vi "BuildDecisionTree_alt.vi"(8 "error in (no error)":errorcluster, 9 "Current Player":T1=enum."Player 1", 10 "Gameboard":T2=[enum."None", enum."None", enum."None", enum."None", enum."None", enum."None", enum."None", enum."None", enum."None"], 11 "DecisionTree In":T3) -> (0 "error out":errorcluster, 2 "Status":T1, 3 "DecisionTree Out":T3)   [LabVIEW 2020]
uses:
  controls/DecisionTree.ctl
  controls/Gameboard Data.ctl
  controls/DecisionTreeRecord.ctl
  controls/Player.ctl
  GetEquivalentKeysNumeric.vi
  AllLines.vi
  MakeSquare.vi
  Flatten2DArray.vi
  <vilib>/Utility/error.llb/Error Cluster From Error Code.vi
  GetAllIsometriesOf2DArray.vi
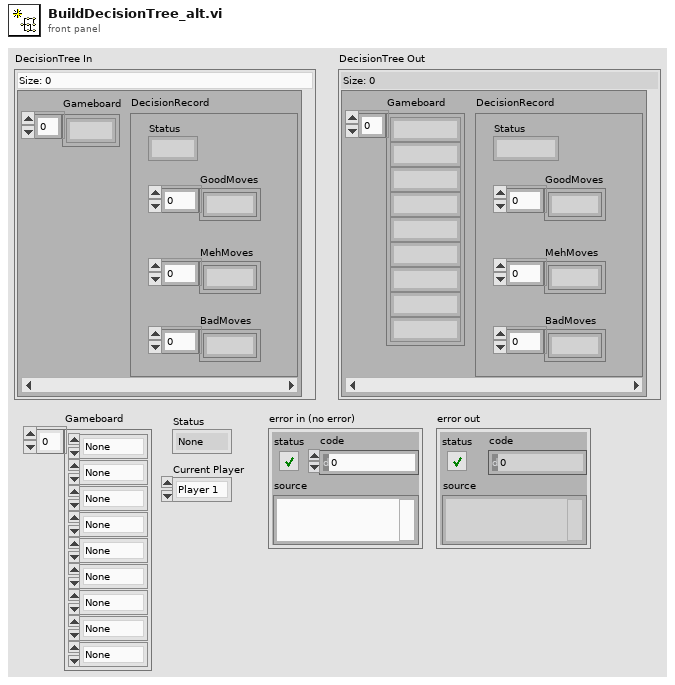
[diagram p1: front panel]
types:
  T1 = typedef "Player.ctl" = enum16{"None", "Player 1", "Player 2"}
  T2 = typedef "Gameboard Data.ctl" = enum16{"None", "Player 1", "Player 2"}[]
  T3 = typedef "DecisionTree.ctl" = map{T2, T4}
  T4 = typedef "DecisionTreeRecord.ctl" = cluster{"Status":T1, "GoodMoves":i8[], "MehMoves":i8[], "BadMoves":i8[]}
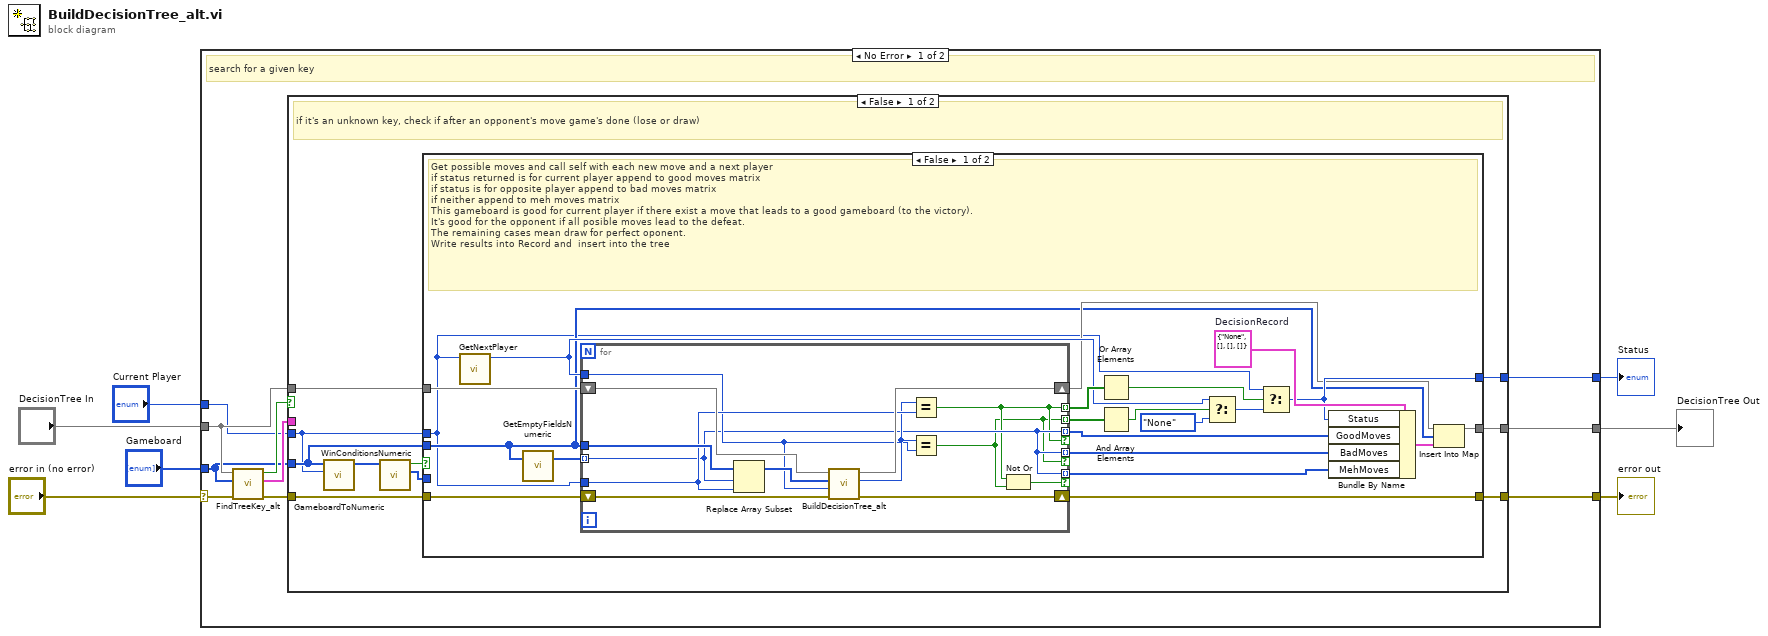
[diagram p0: block diagram]
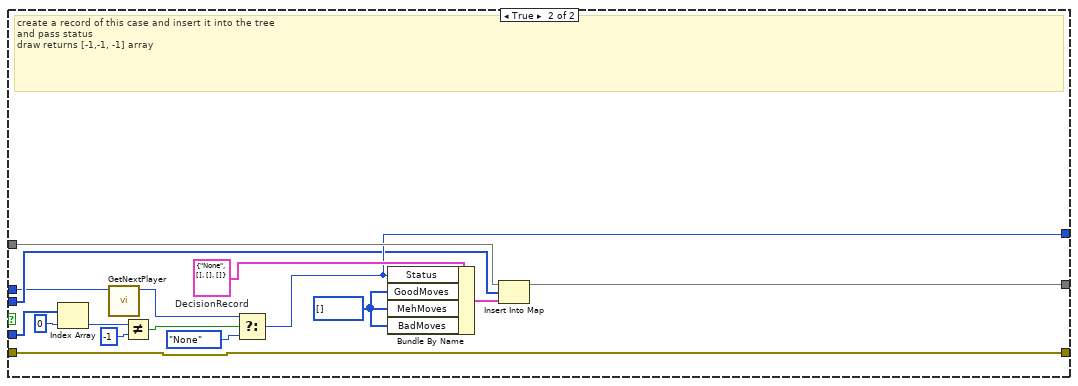
[diagram p2: hidden frame]
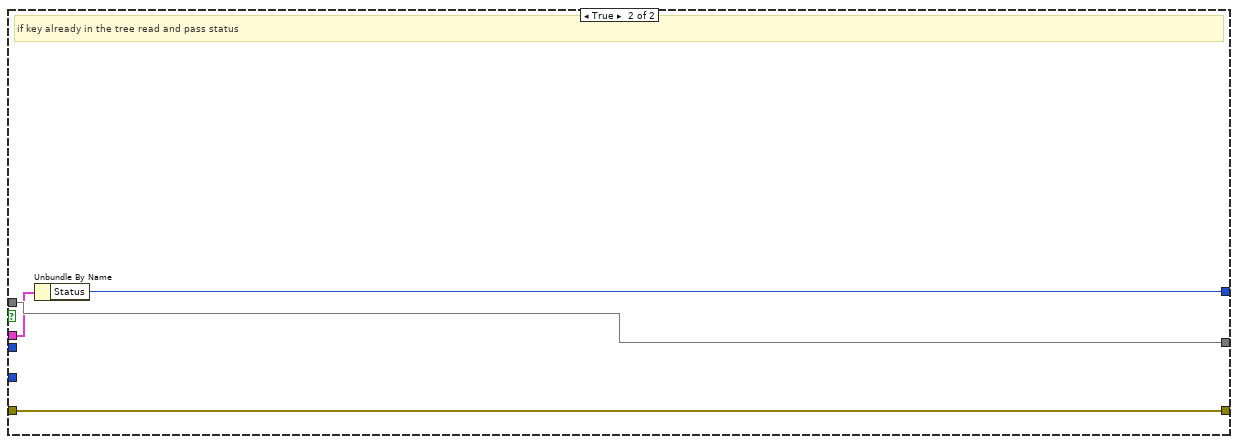
[diagram p3: hidden frame]
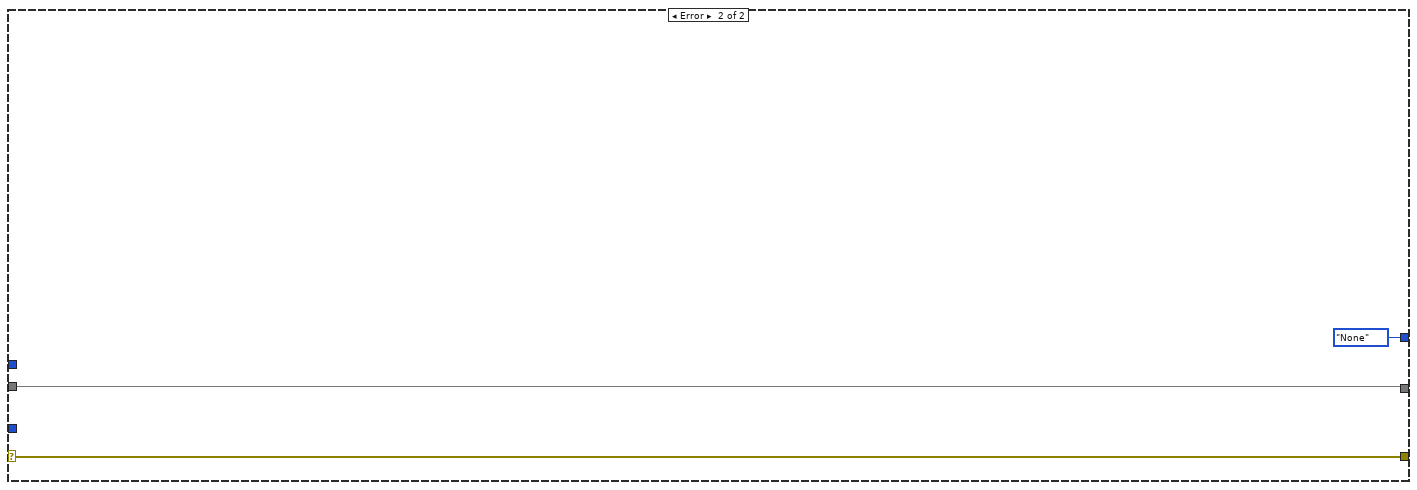
[diagram p4: hidden frame]
diagram:
  n1 = case shown="No Error" "error in (no error)" {
    selector: "error in (no error)" -> [w17 w84]
    tunnel: [w12 w84] -> w6
    tunnel: "Gameboard" -> [w9 _]
    tunnel: "Current Player" -> [w8 _]
    tunnel: [w10 Player."None" ("Status")] -> w3
    tunnel: "DecisionTree In" -> [w14 w82]
    tunnel: [w13 w82] -> w1
    frame No Error {
      # "search for a given key"
      n2 = call "FindTreeKey_alt.vi"("error in (no error)"=w17, "Key"=w9, "Map"=w14) -> ("error out"=w15:errorcluster, "DecisionRecord"=w11:T4, "IsFound?"=w16:bool)  [unwired: 5 in, 1 out]
      n3 = case shown="False" w16 {
        tunnel: w15 -> [w22 w80]
        tunnel: w14 -> [w21 w81]
        tunnel: [w20 w81] -> w13
        tunnel: [w18 w80] -> w12
        tunnel: w11 -> [_ w79]
        tunnel: [w19 w78] -> w10
        tunnel: w9 -> [w24 _]
        tunnel: w8 -> [w23 _]
        frame False {
          # "if it's an unknown key, check if after an opponent's move game's done (lose or draw)"
          n4 = call "GameboardToNumeric.vi"("CurrentPlayer"=w23, "Gameboard"=w24) -> ("NumericGameboard"=w25:i8[])  [unwired: 9 in]
          n5 = call "WinConditionsNumeric.vi"("NumericGameboard"=w25) -> ("LineIndices"=w26:i8[], "End?"=w27:bool)  [unwired: 9 in]
          n6 = case shown="False" w27 {
            tunnel: w26 -> [_ w77]
            tunnel: w24 -> [w29 w67]
            tunnel: w23 -> [w28 w63]
            tunnel: w22 -> [w46 w68]
            tunnel: w21 -> [w47 w72]
            tunnel: [w32 w71] -> w20
            tunnel: [w34 w69] -> w19
            tunnel: [w30 w68] -> w18
            frame False {
              w38 = T4 {"Status"=enum."None", "GoodMoves"=[], "MehMoves"=[], "BadMoves"=[]}  # DecisionRecord
              # "Get possible moves and call self with each new move and a next player\nif status returned is for current player append to good moves matrix\nif status is for opposite player append to bad moves matrix\nif neither append to meh moves matrix\nThis gameboard is good for current player if there exist a move that leads to a good gameboard (to the victory).\nIt's good for the opponent if all posible moves lead to the defeat. \nThe remaining cases mean draw for perfect oponent.\nWrite results into Record and  insert into the tree"
              n7 = call "GetNextPlayer.vi"("current"=w28) -> ("next"=w40:T1)  [unwired: 10 in]
              n8 = call "GetEmptyFieldsNumeric.vi"("NumericGameboard"=w29) -> ("Indices"=w48:i8[])  [unwired: 2 in]
              n9 = for {
                tunnel: w48 -> [w52] mode=indexing
                tunnel: w29 -> [w61]
                tunnel: w28 -> [w55]
                tunnel: w40 -> [w53]
                shift-right: [w57] -> w33
                shift-left: w47 -> [w60]
                shift-right: [w56] -> w30
                shift-left: w46 -> [w58]
                tunnel: [w52] -> w37 mode=indexing if=w50
                tunnel: [w52] -> w36 mode=indexing if=w49
                tunnel: [w52] -> w35 mode=indexing if=w51
                tunnel: [w50] -> w45 mode=indexing
                tunnel: [w49] -> w44 mode=indexing
                n10 = Replace Array Subset(array=w61, new element=w55, index=w52) -> (w59:T2)
                n11 = call "BuildDecisionTree_alt.vi"("error in (no error)"=w58, "Current Player"=w53, "Gameboard"=w59, "DecisionTree In"=w60) -> ("error out"=w56:errorcluster, "Status"=w54:T1, "DecisionTree Out"=w57:T3)  [unwired: 5 in]
                n12 = Equal?(x=w54, y=w55) -> (x = y?=w50:bool)
                n13 = Equal?(x=w54, y=w53) -> (x = y?=w49:bool)
                n14 = Not Or(1:w49, 2:w50) -> (0:w51:bool)
              }
              n15 = Or Array Elements(Boolean array=w45) -> (logical OR=w43:bool)
              n16 = And Array Elements(Boolean array=w44) -> (logical AND=w41:bool)
              n17 = Select(t=w40, s=w41, f=Player."None") -> (s? t:f=w42:T1)
              n18 = Select(t=w28, s=w43, f=w42) -> (s? t:f=w34:T1)
              n19 = Bundle By Name(cluster=w38, "Status"=w34, "GoodMoves"=w37, "BadMoves"=w36, "MehMoves"=w35) -> (w31:T4)
              n20 = Insert Into Map(map in=w33, key=w29, value=w31) -> (map out=w32:T3)  [unwired: 2 out]
            }
            frame True {
              w66 = i8[] [] ("GoodMoves")
              w73 = T4 {"Status"=enum."None", "GoodMoves"=[], "MehMoves"=[], "BadMoves"=[]}  # DecisionRecord
              # "create a record of this case and insert it into the tree\nand pass status\ndraw returns [-1,-1, -1] array"
              n21 = Index Array(array=w77, index=0) -> (element=w64:i8)
              n22 = call "GetNextPlayer.vi"("current"=w63) -> ("next"=w62:T1)  [unwired: 10 in]
              n23 = Not Equal?(x=w64, y=i8 -1) -> (x != y?=w75:bool)
              n24 = Select(t=w62, s=w75, f=Player."None") -> (s? t:f=w69:T1)
              n25 = Bundle By Name(cluster=w73, "Status"=w69, "GoodMoves"=w66, "MehMoves"=w66, "BadMoves"=w66) -> (w70:T4)
              n26 = Insert Into Map(map in=w72, key=w67, value=w70) -> (map out=w71:T3)  [unwired: 2 out]
            }
          }
        }
        frame True {
          # "if key already in the tree read and pass status"
          n27 = Unbundle By Name(w79) -> ("Status"=w78:T1)
        }
      }
    }
    frame Error {
    }
  }
  "DecisionTree Out" <- w1
  "error out" <- w6
  "Status" <- w3
